vi "Adapt Waveform.vi"(8 "Error":errorcluster, 9 "Waveform":T1, 11 "(WavBuf)":refnum<class "(WavBuf).lvclass">) -> (0 "Error Out":errorcluster, 1 "Waveform Out":T1, 3 "(WavBuf) Out":refnum<class "(WavBuf).lvclass">)   [LabVIEW 2016, in "(WavBuf).lvclass"]
uses:
  (WavBuf).lvclass
  Universal Controls/Waveform_Data.ctl
  (WavBuf).lvclass/(WavBuf).ctl
  Support/Measure_Decimate Dbl Array.vi
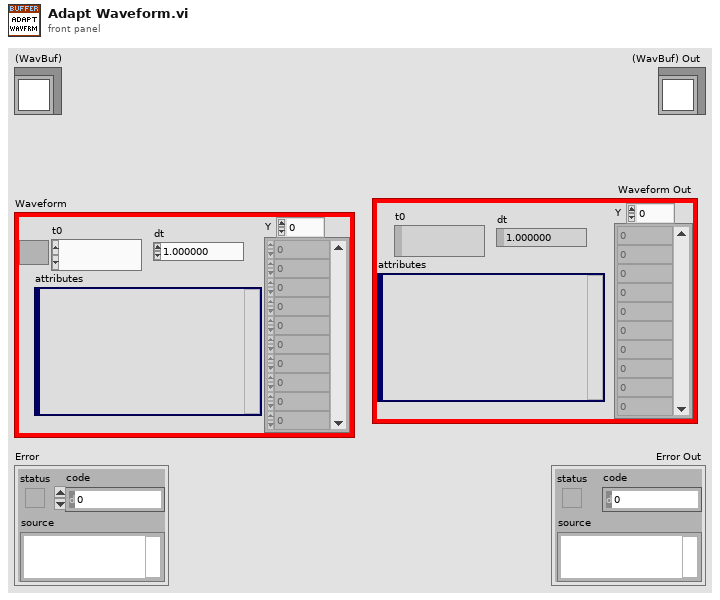
[diagram p1: front panel]
types:
  T1 = typedef "Waveform_Data.ctl" = waveform(dbl)
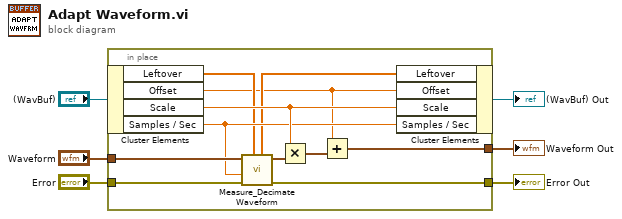
[diagram p0: block diagram]
diagram:
  n1 = in-place {
    in-place-border: [w8] -> w6
    in-place-border: [w11] -> w5
    in-place-border: "Waveform" -> [w16]
    in-place-border: "Error" -> [w12]
    n2 = in-place-cluster #1("(WavBuf)") -> ("Leftover"=w14:dbl[], "Offset"=w7:dbl, "Scale"=w17:dbl, "Samples / Sec"=w15:dbl)
    n3 = call "Measure_Decimate Waveform.vi"("Leftover last"=w14, "Error"=w12, "Target Sample Rate"=w15, "Waveform To Decimate"=w16) -> ("Error Out"=w11:errorcluster, "Waveform Out"=w10:T1, "Leftover Out"=w13:dbl[])  [unwired: 5 in]
    n4 = Multiply(x=w17, y=w10) -> (x*y=w9:T1)
    n5 = Add(x=w7, y=w9) -> (x+y=w8:T1)
    n6 = in-place-cluster #1("Leftover"=w13, "Offset"=w7, "Scale"=w17, "Samples / Sec"=w15) -> (→"(WavBuf) Out":refnum<class "(WavBuf).lvclass">)
  }
  "Waveform Out" <- w6
  "Error Out" <- w5
